vi "SSC DCPower Force Current Array Symmetric Limits.vi"(0 "DCPower SSC in":T1[](array[typedef]), 1 "Current Level Range (A)":dbl[](array[numeric]) format="%#_6p", 2 "Voltage Limit Range (V)":dbl[](array[numeric]) format="%#_6p", 5 "Current Level (A)":dbl[](array[numeric]) format="%#_6p", 7 "Voltage Limit (V)":dbl[](array[numeric]) format="%#_6p", 11 "error in":errorcluster) -> (4 "DCPower SSC out":T1[](array[typedef]), 15 "error out":errorcluster)   [LabVIEW 2020]
doc: "This VI forces current on the provided sessions.\n\nAll input arrays need to be populated with a value for each session, or else the for loop won't iterate for all sessions."
uses:
  SSC DCPower.ctl
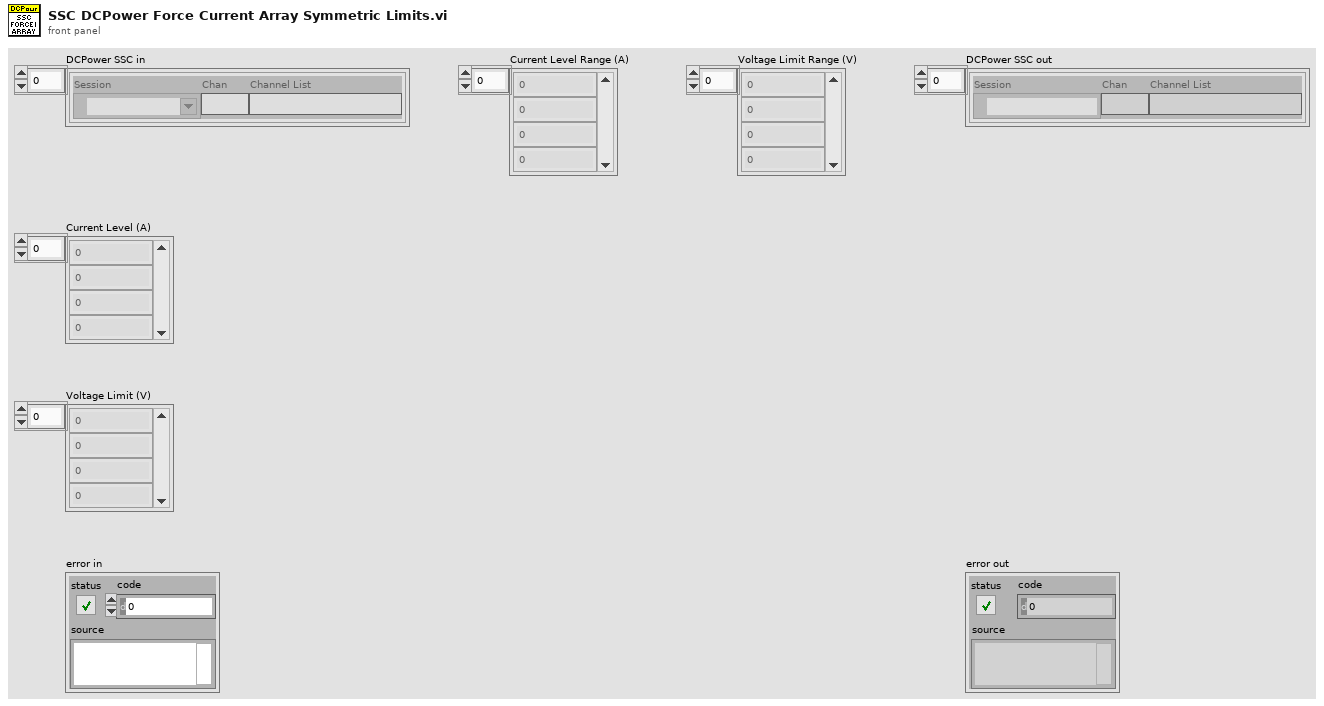
[diagram p1: front panel]
types:
  T1 = typedef "SSC DCPower.ctl" = cluster{"Session":refnum<k15>, "Chan":string, "Channel List":string}
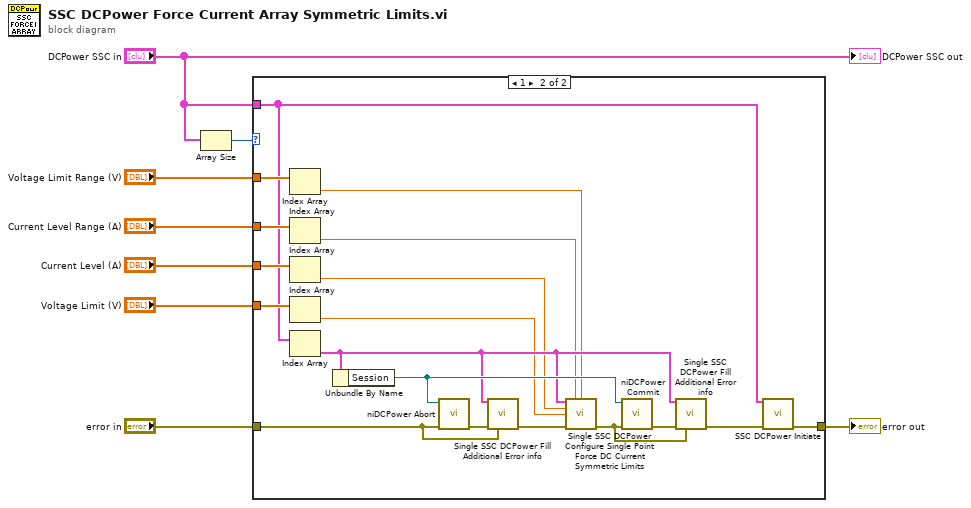
[diagram p0: block diagram]
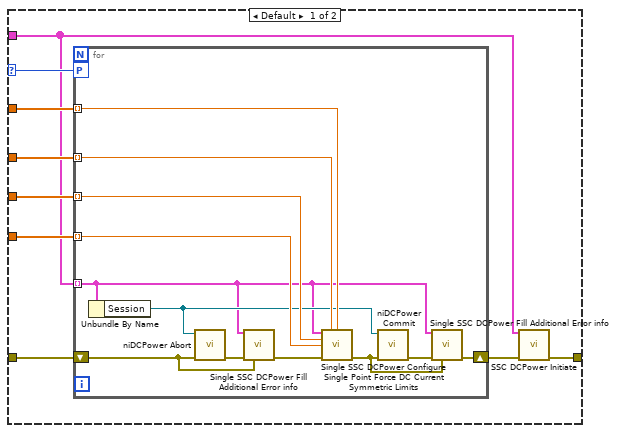
[diagram p2: hidden frame]
diagram:
  n1 = Array Size(array="DCPower SSC in") -> (size(s)=w8:i32)
  n2 = case shown="1" w8 {
    selector: w8 -> [w17 _]
    tunnel: "Current Level (A)" -> [w16 w47]
    tunnel: "Voltage Limit (V)" -> [w15 w46]
    tunnel: "Current Level Range (A)" -> [w14 w45]
    tunnel: [w12 w43] -> w4
    tunnel: "error in" -> [w11 w42]
    tunnel: "Voltage Limit Range (V)" -> [w10 w41]
    tunnel: "DCPower SSC in" -> [w9 w40]
    frame Default {
      n3 = for {
        workers-P: w17 -> [_]
        tunnel: w9 -> [w20] mode=indexing
        tunnel: w16 -> [w29] mode=indexing
        tunnel: w15 -> [w28] mode=indexing
        tunnel: w14 -> [w27] mode=indexing
        tunnel: w10 -> [w26] mode=indexing
        shift-right: [w21] -> w13
        shift-left: w11 -> [w19]
        n4 = Unbundle By Name(w20) -> ("Session"=w23:refnum<k15>)
        n5 = call <instrlib>:"niDCPower Abort.vi"("error in (no error)"=w19, "instrument handle"=w23) -> ("error out"=w25:errorcluster)  [unwired: 8 in, 1 out]
        n6 = call "Single SSC DCPower Fill Additional Error info.vi"("DCPower SSC in"=w20, "error in"=w25, "previous error in"=w19) -> ("error out"=w22:errorcluster)  [unwired: 12 in]
        n7 = call "Single SSC DCPower Configure Single Point Force DC Current Symmetric Limits.vi"("DCPower SSC in"=w20, "Current Level Range (A)"=w27, "Voltage Limit Range (V)"=w26, "Current Level (A)"=w29, "Voltage Limit (V)"=w28, "error in"=w22) -> ("error out"=w18:errorcluster)  [unwired: 8 in, 1 out]
        n8 = call <instrlib>:"niDCPower Commit.vi"("error in (no error)"=w18, "instrument handle"=w23) -> ("error out"=w24:errorcluster)  [unwired: 8 in, 1 out]
        n9 = call "Single SSC DCPower Fill Additional Error info.vi"("DCPower SSC in"=w20, "error in"=w24, "previous error in"=w18) -> ("error out"=w21:errorcluster)  [unwired: 12 in]
      }
      n10 = call "SSC DCPower Initiate.vi"("DCPower SSC in"=w9, "error in"=w13) -> ("error out"=w12:errorcluster)  [unwired: 12 in, 1 out]
    }
    frame 1 {
      n11 = Index Array(array=w41) -> (element=w33:dbl)  [unwired: 1 in]
      n12 = Index Array(array=w45) -> (element=w32:dbl)  [unwired: 1 in]
      n13 = Index Array(array=w47) -> (element=w31:dbl)  [unwired: 1 in]
      n14 = Index Array(array=w46) -> (element=w30:dbl)  [unwired: 1 in]
      n15 = Index Array(array=w40) -> (element=w34:T1)  [unwired: 1 in]
      n16 = Unbundle By Name(w34) -> ("Session"=w37:refnum<k15>)
      n17 = call <instrlib>:"niDCPower Abort.vi"("error in (no error)"=w42, "instrument handle"=w37) -> ("error out"=w39:errorcluster)  [unwired: 8 in, 1 out]
      n18 = call "Single SSC DCPower Fill Additional Error info.vi"("DCPower SSC in"=w34, "error in"=w39, "previous error in"=w42) -> ("error out"=w36:errorcluster)  [unwired: 12 in]
      n19 = call "Single SSC DCPower Configure Single Point Force DC Current Symmetric Limits.vi"("DCPower SSC in"=w34, "Current Level Range (A)"=w32, "Voltage Limit Range (V)"=w33, "Current Level (A)"=w31, "Voltage Limit (V)"=w30, "error in"=w36) -> ("error out"=w35:errorcluster)  [unwired: 8 in, 1 out]
      n20 = call <instrlib>:"niDCPower Commit.vi"("error in (no error)"=w35, "instrument handle"=w37) -> ("error out"=w38:errorcluster)  [unwired: 8 in, 1 out]
      n21 = call "Single SSC DCPower Fill Additional Error info.vi"("DCPower SSC in"=w34, "error in"=w38, "previous error in"=w35) -> ("error out"=w44:errorcluster)  [unwired: 12 in]
      n22 = call "SSC DCPower Initiate.vi"("DCPower SSC in"=w40, "error in"=w44) -> ("error out"=w43:errorcluster)  [unwired: 12 in, 1 out]
    }
  }
  "error out" <- w4
  "DCPower SSC out" <- "DCPower SSC in"
